vi "Query Output ALC State.vi"(8 "error in (no error)":errorcluster, 10 "Platform Slot Number (10)":i16=10 min=-1 max=255, 11 "VISA resource name":refnum<visa-resource-name>) -> (0 "error out":errorcluster, 2 "Automatic Leveling Control Enabled":bool, 3 "VISA resource name out":refnum<visa-resource-name>)   [LabVIEW 2018, in "LTB-1.lvlib" / "3150.lvlib"]
doc: "Output indicates if the power tracking that controls the output power level has been activated or not. The power tracking is done via the ALC (Automatic Leveling Control) loop.\n\n<B>Note:</B>\nThis command is applicable only for <B>Self-adjusting module</B> type of 3150. For standard module, \"Power control option not available.\" message will be returned as it doesn't support Output Power control mode. Refer IQS-3150 user manual for more information."
uses:
  3150.lvlib
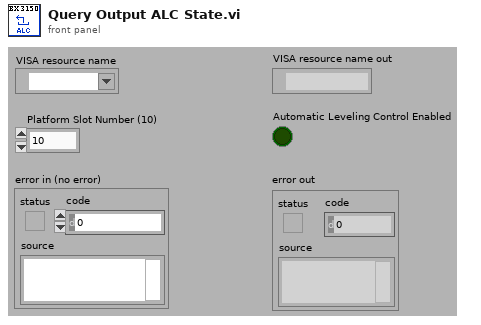
[diagram p1: front panel]
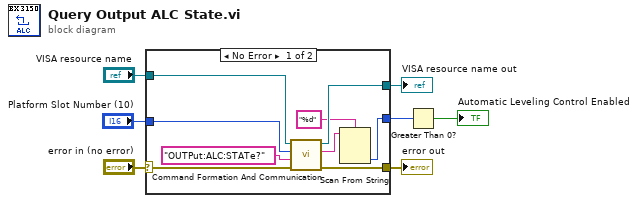
[diagram p0: block diagram]
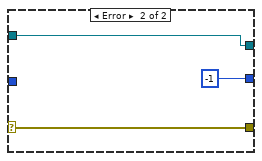
[diagram p2: hidden frame]
diagram:
  n1 = case shown="No Error" "error in (no error)" {
    selector: "error in (no error)" -> [w15 w18]
    tunnel: "VISA resource name" -> [w16 w19]
    tunnel: [w14 w19] -> w5
    tunnel: [w13 w18] -> w4
    tunnel: [w9 -1] -> w2
    tunnel: "Platform Slot Number (10)" -> [w8 _]
    frame No Error {
      n2 = call "Command Formation And Communication.vi"("error in (no error)"=w15, "Command"="OUTPut:ALC:STATe?", "Platform Slot Number"=w8, "VISA resource name"=w16) -> ("error out"=w13:errorcluster, "Response"=w10:string, "VISA resource name out"=w14:refnum<visa-resource-name>)  [unwired: 5 out]
      n3 = Scan From String(format string="%d", input string=w10) -> (output 1=w9:i32)  [unwired: 2 in, 4 out]
    }
    frame Error {
    }
  }
  "VISA resource name out" <- w5
  "error out" <- w4
  n4 = Greater Than 0?(x=w2) -> (x > 0?=→"Automatic Leveling Control Enabled":bool)
